vi "Arm Up-Down.vi"(11 "Robot Comands":T1) -> ()   [LabVIEW 2014]
uses:
  Joystick/Robot Commands.ctl
  <vilib>/Rock Robotics/WPI/Relay/WPI_RelayValue.ctl
  Global Variables/Global Variables.vi
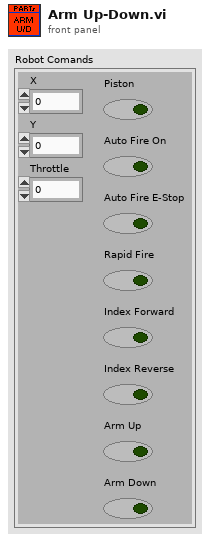
[diagram p1: front panel]
types:
  T1 = typedef "Robot Commands.ctl" = cluster{"X":dbl, "Y ":dbl, "Throttle":dbl, "Piston":bool, "Auto Fire On":bool, "Auto Fire E-Stop":bool, "Rapid Fire":bool, "Index Forward":bool, "Index Reverse ":bool, "Arm Up":bool, "Arm Down":bool}
  T2 = typedef "WPI_RelayValue.ctl" = enum16{"Off", "On", "Forward", "Reverse"}
  T3 = typedef "WPI_RelayDevRef.ctl" = cluster{"DevStatus":errorcluster, "Relay Channel":T4, "Controller":T5, "Relay Direction":T6}
  T4 = typedef "FPGA_DIORelayChannel.ctl" = enum8{"Relay 0", "Relay 1", "Relay 2", "Relay 3", "Invalid"}
  T5 = typedef "FPGA_TypedefDigitalModule.ctl" = enum16{"Controller 1"}
  T6 = typedef "WPI_RelayDirection.ctl" = enum16{"Both directions", "Forward only", "Reverse only"}
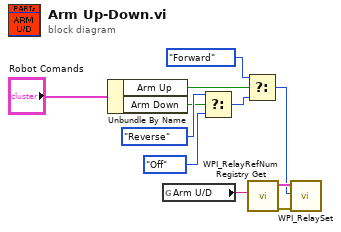
[diagram p0: block diagram]
diagram:
  n1 = Unbundle By Name("Robot Comands") -> ("Arm Up"=w3:bool, "Arm Down"=w2:bool)
  n2 = global read "Global Variables.vi" "Arm U/D"() -> (w9:string)
  n3 = Select(t=WPI_RelayValue."Reverse" ("RelayValue"), s=w2, f=WPI_RelayValue."Off" ("RelayValue")) -> (s? t:f=w5:T2)
  n4 = Select(t=WPI_RelayValue."Forward" ("RelayValue"), s=w3, f=w5) -> (s? t:f=w1:T2)
  n5 = call <vilib>:"WPI_RelayRefNum Registry Get.vi"("refnum name"=w9) -> ("error out"=w10:errorcluster, "RelayDevRef"=w11:T3)  [unwired: 9 in]
  n6 = call <vilib>:"WPI_RelaySet.vi"("error in (no error)"=w10, "RelayValue"=w1, "RelayDevRef"=w11) -> ()  [unwired: 7 in, 2 out]
